vi "Read Curvatures.vi"(8 "error in (no error)":errorcluster, 11 "EdgeDetectionProcessor in":refnum<class "EdgeDetectionProcessor.lvclass">) -> (0 "error out":errorcluster, 2 "Curvatures":T1[](array[typedef]), 3 "EdgeDetectionProcessor out":refnum<class "EdgeDetectionProcessor.lvclass">)   [LabVIEW 2018, in "EdgeDetectionProcessor.lvclass"]
uses:
  EdgeDetectionProcessor.lvclass
  private/Curvature Data STYP.ctl
  EdgeDetectionProcessor.lvclass/EdgeDetectionProcessor.ctl
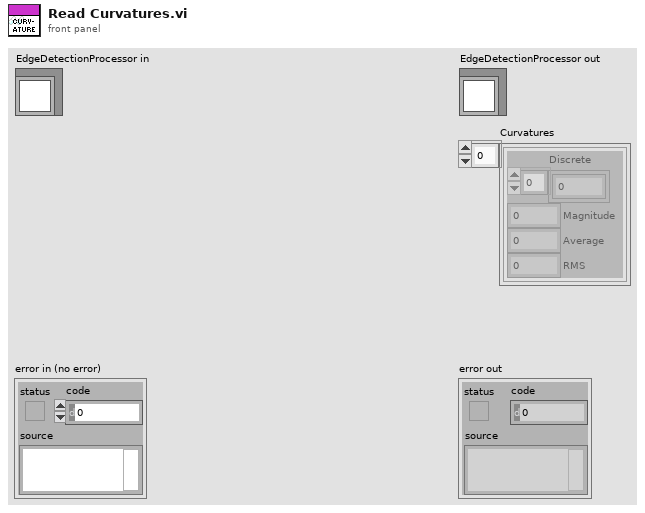
[diagram p1: front panel]
types:
  T1 = typedef "EdgeDetectionProcessor.lvclass/Curvature Data STYP.ctl" = cluster{"Discrete":dbl[], "Magnitude":dbl, "Average":dbl, "RMS":dbl}
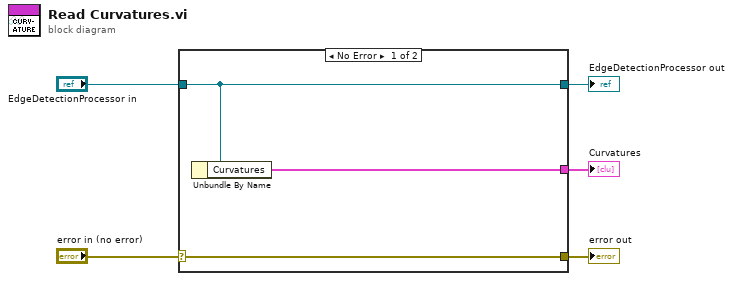
[diagram p0: block diagram]
diagram:
  n1 = case shown="No Error" "error in (no error)" {
    selector: "error in (no error)" -> [w8 w9]
    tunnel: [w8 w9] -> w4
    tunnel: [w7 w10] -> w2
    tunnel: "EdgeDetectionProcessor in" -> [w7 w10]
    tunnel: [w6 _] -> w1
    frame No Error {
      n2 = Unbundle By Name(w7) -> ("Curvatures"=w6:T1[])
    }
    frame Error {
    }
  }
  "error out" <- w4
  "EdgeDetectionProcessor out" <- w2
  "Curvatures" <- w1
